vi "Create Layer from Image.vi"(6 "Layer type":T2, 8 "error in":errorcluster, 9 "Monochrome Data in":T1, 10 "Color Data In":T1, 11 "LayerName":string) -> (0 "error out":errorcluster, 2 "Layer.lvclass out":refnum<class "Layer.lvclass">)   [LabVIEW 2020, in "lv_icon.lvlib"]
doc: "Create a User Layer from the Image Data"
uses:
  <vilib>/LabVIEW Icon API/lv_icon/lv_icon.lvlib
  <vilib>/LabVIEW Icon API/lv_icon/Classes/Layer/Layer.lvclass
  <vilib>/picture/picture.llb/imagedata.ctl
  <vilib>/LabVIEW Icon API/lv_icon/Controls/LayerType.ctl
  <vilib>/LabVIEW Icon API/lv_icon/Controls/Layer.ctl
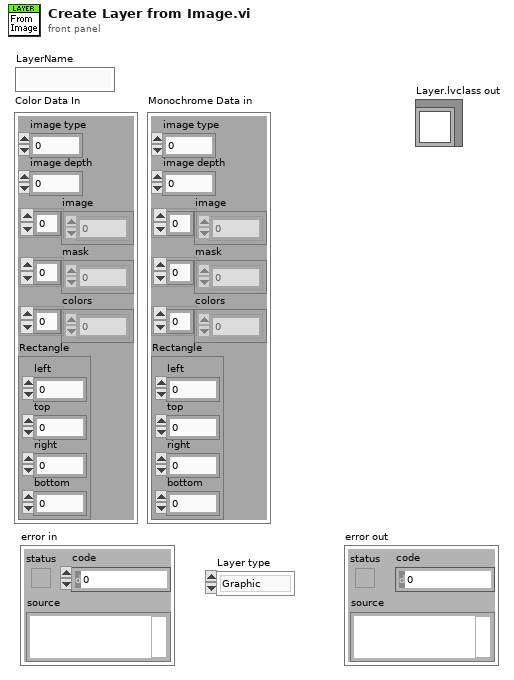
[diagram p1: front panel]
types:
  T1 = typedef "imagedata.ctl" = cluster{"image type":i32, "image depth":i32, "image":u8[], "mask":u8[], "colors":u32[], "Rectangle":cluster{"left":i16, "top":i16, "right":i16, "bottom":i16}}
  T2 = typedef "LayerType.ctl" = enum16{"Graphic", "Text", "Tool", "Graphic Drop"}
  T3 = typedef "Layer.ctl" = cluster{"LayerIcon":picture, "LayerName":string, "Opacity":u8, "Visibility?":bool}
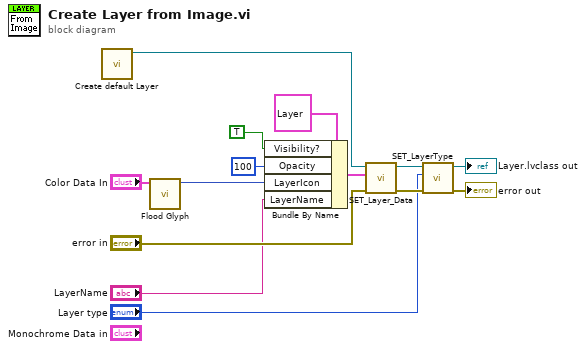
[diagram p0: block diagram]
diagram:
  n1 = call <vilib>:"Create default Layer.vi"() -> ("Layer.lvclass out"=w1:refnum<class "Layer.lvclass">)  [unwired: 1 in, 10 out]
  n2 = call <vilib>:"Flood Glyph.vi"("image data"="Color Data In") -> ("Pic Out"=w6:picture)  [unwired: 1 in, 9 out]
  n3 = Bundle By Name(cluster=T3 {"LayerIcon"=bytes[0], "LayerName"="", "Opacity"=0, "Visibility?"=FALSE} ("Data"), "Visibility?"=TRUE, "Opacity"=u8 100, "LayerIcon"=w6, "LayerName"="LayerName") -> (w9:T3)
  n4 = call-dynamic "SET_Layer_Data.vi"("error in (no error)"="error in", "Data"=w9, "Layer.lvclass in"=w1) -> ("error out"=w11:errorcluster, "Layer.lvclass out"=w8:refnum<class "Layer.lvclass">)  [unwired: 1 in, 6 out]
  n5 = call-dynamic "SET_LayerType.vi"("error in (no error)"=w11, "Type"="Layer type", "Layer.lvclass in"=w8) -> ("error out"=→"error out":errorcluster, "Layer.lvclass out"=→"Layer.lvclass out":refnum<class "Layer.lvclass">)  [unwired: 7 out]
